vi "Dashboard Main.vi"() -> ()   [LabVIEW 2016]
uses:
  Program Files/National Instruments/LabVIEW 2016/examples/FRC/roboRIO/Vision/2017 Vision Example/Vision Support Code/Camera Types.ctl
  <vilib>/Rock Robotics/Network Tables/NT Read Boolean.vi
  <vilib>/Rock Robotics/Network Tables/NT Write Number.vi
  <vilib>/Rock Robotics/Network Tables/NT Read Number.vi
  <vilib>/Utility/file.llb/Read Delimited Spreadsheet (DBL).vi
  <vilib>/Utility/file.llb/Write Delimited Spreadsheet (DBL).vi
  <vilib>/vision/NI_Vision_Development_Module.lvlib
panel:
  out "Original Image":T1(plugin-control)
  in  "Dashboard Tab":T2(tab)=enum."\"Fudge\" Variables"
  out "Trim Close":dbl=-1.0
  out "Trim Far":dbl=-1.0
  out "Have Gear?":bool
  out "Drive Mode":bool
  in  "Auto Selector":T3(ring)
  out "Aimed?":bool
  out "IR Distance":bool
  out "Mode":T4(ring)=enum."Auto Disabled"
  in  "Camera Name":string(combo)="No Camera Selection"
  out "Camera Info":cluster{"Mbps LED":bool, "Mbps":dbl, "fps":dbl} {"fps" format="%#.1g"; "Mbps" format="%#.1g"}
  in  "Camera Type":T5=enum."MS HD3000 square"
  in  "LED Color":T6={"Hue"={70.0, 130.0}, "Sat"={150.0, 255.0}, "Val"={100.0, 255.0}} {"Hue" scale=0.0..255.0 scale format="%#_3g"}
  in  "Annotate":bool=TRUE
  in  "Color Mode":u16(ring)=2 items=["RGB", "HSL", "HSV", "HSI"]
  in  "Particles":dbl=4.0
  in  "Score Cutoff %":dbl=75.0
  out "Qualified Particles":i32
  in  "Std Devs for Calibration":cluster{"H":dbl, "S":dbl, "V":dbl}={"H"=4.0, "S"=6.0, "V"=6.0}
  in  "Line Border":cluster{"Top":dbl, "Bottom":dbl}={"Top"=6.0, "Bottom"=1.0}
  in  "Camera Settings":T7={"Frame Rate"=30, "Compression"=30, "Size"=1, "DB Camera Config"=FALSE} {"Frame Rate" scale=1.0..30.0; "Compression" scale=100.0..-1.0; "Size" items=["640x480", "320x240", "160x120"]}
  out "Mask":T1(plugin-control)
  out "Results":T8 {"Score" format="%#_3g"; "Pixels"."Rectangle"."Numeric 5" format="%#_3g"; "Pixels"."Rectangle"."Numeric 3" format="%#_3g"; "Pixels"."Rectangle"."Numeric 2" format="%#_3g"; "Pixels"."Rectangle"."Numeric" format="%#_3g"; "Normalized"."Rectangle"."Numeric 5" format="%#_2g"; "Normalized"."Rectangle"."Numeric 3" format="%#_2g"; "Normalized"."Rectangle"."Numeric 2" format="%#_2g"; "Normalized"."Rectangle"."Numeric" format="%#_2g"; "Normalized"."Center"."?" format="%#_3g"; "Normalized"."Center"."?" format="%#_3g"; "Distance (ft)" format="%#_3g"}
  in  "Autoaim fast":dbl=0.25
  in  "Autoaim mid":dbl=0.2
  in  "Autoaim slow":dbl=0.19
  in  "FF B40":dbl=0.7
  in  "B40yDepth":dbl=62.0
  in  "center gear depth":dbl=31.0
  in  "FF B10 G":dbl=0.72
  in  "FF R60 P1":dbl=0.71
  in  "FF R60 P2":dbl=0.704
  in  "Hopper Close":dbl=0.6
  in  "Hopper Far":dbl=0.75
  in  "R60P2yDepth":dbl=-74.0
  in  "R60P1yDepth":dbl=-60.0
  in  "Camera Target":dbl=0.06
  in  "FF Far Tele":dbl=0.7
  in  "FF Close Tele":dbl=0.66
  in  "Intake Speed":dbl=0.8
  out "Path":path
  out "Tree":string(tree)
  out "NT Connection":bool
  in  "Select Auto":string(combo)="Select Autonomous ..."
  out "Background":bool
  in  "TCP":refnum<k5>
  out "Robot IP":string
  out "Camera Image":T1(plugin-control)
  # "REALLY IMPORTANT"
  # "HW"
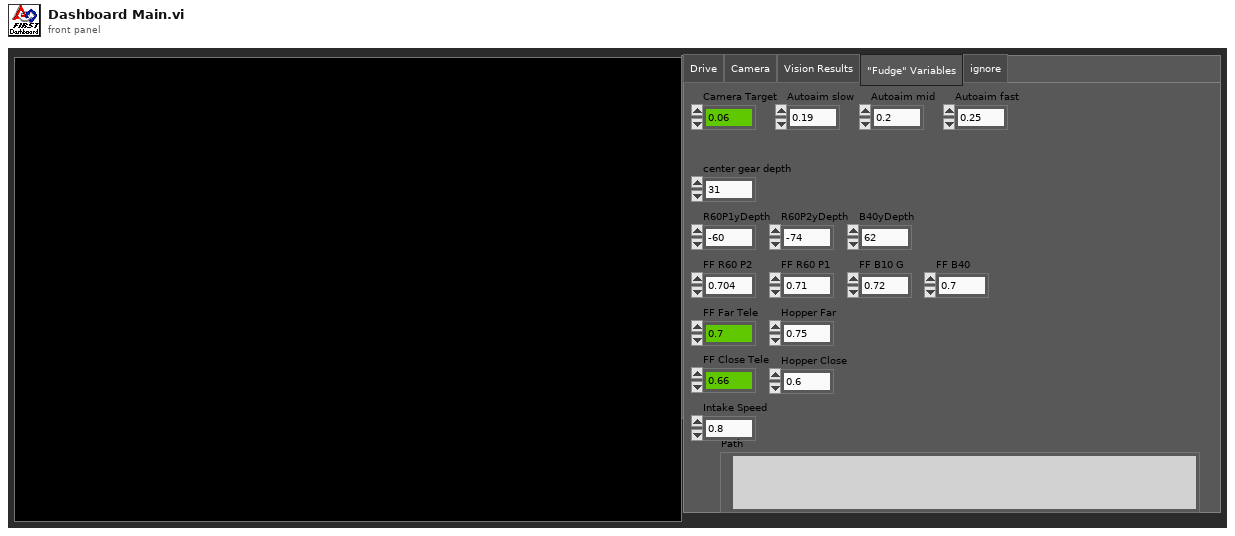
[diagram p1: front panel]
types:
  T1 = typedef "IMAQ Image.ctl" = refnum<image>
  T2 = enum32{"Drive", "Camera", "Vision Results", "\"Fudge\" Variables", "ignore"}
  T3 = enum16{"Do Nothing", "Blue 10 + Gear middle", "Red 10 + Gear middle", "Straight Gear", "Blue 40 P1", "Red 40 P1", "Red 40 P2", "Red 40 + Gear P2 (god auto DNE)", "Blue Side Gear P2 (unproven)"}
  T4 = enum8{"Tele-Op Disabled", "Tele-Op Enabled", "Auto Disabled", "Auto Enabled", "Test Disabled", "Test Enabled", "Disconnected", "No Code", "E-Stop"}
  T5 = typedef "Camera Types.ctl" = enum16{"206", "1011", "1013", "MS HD3000 square", "MS HD3000 640x480"}
  T6 = cluster{"Hue":cluster{dbl, dbl}, "Sat":cluster{dbl, dbl}, "Val":cluster{dbl, dbl}}
  T7 = cluster{"Frame Rate":i32, "Compression":i32, "Size":u16, "DB Camera Config":bool}
  T8 = cluster{"Distance (ft)":dbl, "Score":dbl, "Normalized":cluster{"Center":cluster{dbl, dbl}, "Rectangle":cluster{"Numeric":dbl, "Numeric 2":dbl, "Numeric 3":dbl, "Numeric 5":dbl}}, "Pixels":cluster{"Center":cluster{dbl, dbl}, "Rectangle":cluster{"Numeric":dbl, "Numeric 2":dbl, "Numeric 3":dbl, "Numeric 5":dbl}}}
  T9 = typedef "Particle Parameters" = i32
  T10 = typedef "Image Type" = u32
  T11 = enum32{"Drive", "Basic", "Custom", "Test", "Checklist", "Variables"}
  T12 = cluster{cluster{"Numeric":dbl, "Numeric":dbl}, cluster{"Numeric":dbl, "Numeric":dbl}, cluster{"Numeric":dbl, "Numeric":dbl}}
  T13 = cluster{"Camera Image":refnum<vi>, "Dashboard Tab":refnum<vi>, "Background":refnum<vi>, "Tree":refnum<vi>, "Camera Settings":refnum<vi>, "Camera Name":refnum<vi>, "Camera Info":refnum<vi>}
  T14 = cluster{"Error Strings":string, "Disable Counts":cluster{u16, u16}, "Rail Faults":cluster{u16, u16, u16}, "Robot IP":string, "DB Mode":u8, "Event Info":cluster{"Name":string, "Type":u8, "Number":u16, "Replay":u8}}
  T15 = cluster{"Storage":cluster{"Disk Free":u64, "RAM Block":u32, "RAM free":u32}, "CPU Utilization":cluster{"CPU % ISR":sgl, "CPU % Time Crit":sgl, "CPU % Timed Str":sgl, "CPU % High":sgl, "CPU % Above":sgl, "CPU % Normal":sgl, "CPU % Low":sgl}, "CAN":cluster{"% Bus Utilization":sgl, "Bus Off Cnt":u32, "TX_FIFO Full Cnt":u32, "Receive Error Cnt":u8, "Transmit Error Cnt":u8}, "HID":cluster{"HID Outputs":u32, "Rumble Low":u16, "Rumble High":u16}[]}
  T16 = cluster{"Status bits":cluster{"Test Mode":bool, "Autonomous":bool, "Enabled":bool, "Code Start":bool, "Brownout":bool, "Reserved 2":bool, "Reserved 3":bool, "E-Stop":bool}, "Code Trace":cluster{"Disabled":bool, "TeleOp":bool, "Auto":bool, "Test":bool}, "Controller Type":enum16{"unknown", "cRIO", "roboRio"}, "Code?":enum16{"unknown", "noCode", "code"}, "Battery V":dbl}
  T17 = cluster{"Control Bits":cluster{"TestMode":bool, "Autonomous":bool, "Enabled":bool, "FMS Present":bool, bool, bool, bool, "E-Stop":bool}, "Team Station ":u8, "Countdown":sgl, "Joystick Values":cluster{"Axes":dbl[], "Buttons":bool[], "POVs":i16[]}[]}
  T18 = cluster{"Shift":bool, "Ctrl":bool, "Alt":bool, "Cmd":bool, "Opt":bool}
  T19 = cluster{cluster{dbl, dbl}, cluster{dbl, dbl}, cluster{dbl, dbl}}
  T20 = cluster{"Left":dbl, "Top":dbl, "Right":dbl, "Bottom":dbl}
  T21 = cluster{"Center":cluster{dbl, dbl}, "Rectangle":cluster{"Numeric":dbl, "Numeric 2":dbl, "Numeric 3":dbl, "Numeric 5":dbl}}
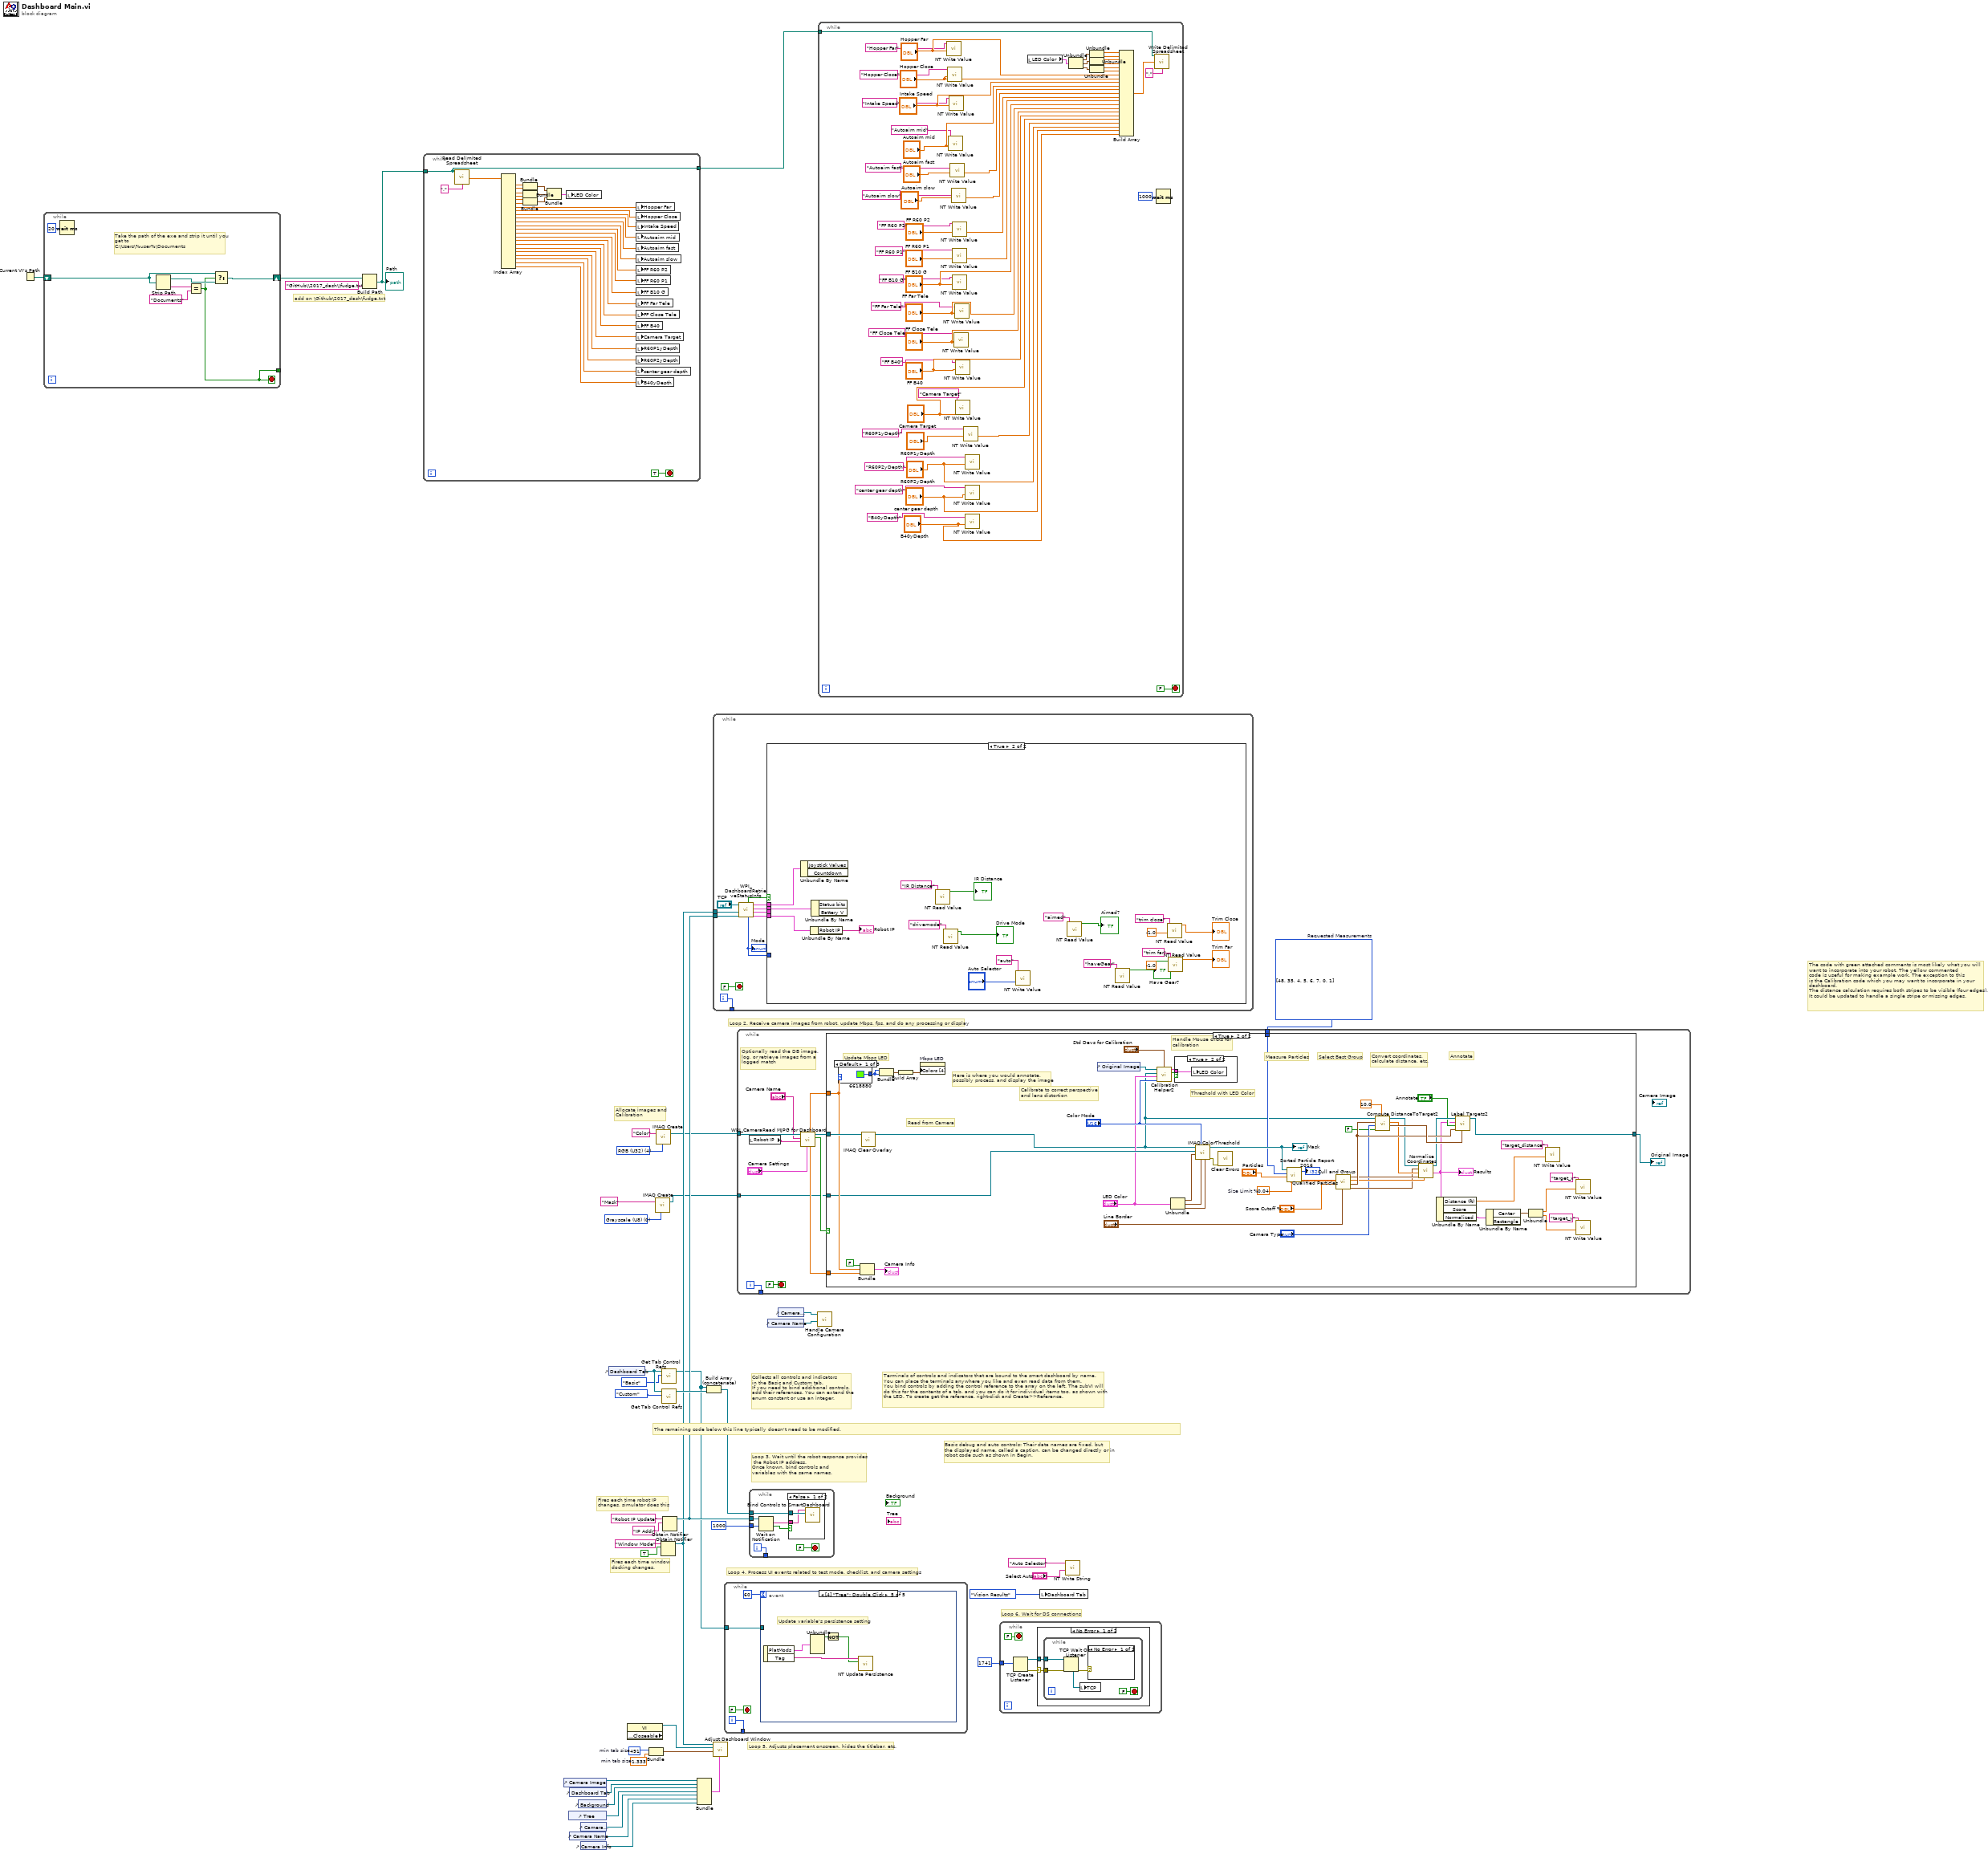
[diagram p0: block diagram]
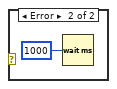
[diagram p2: hidden frame]
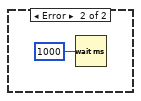
[diagram p3: hidden frame]
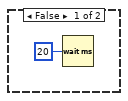
[diagram p4: hidden frame]
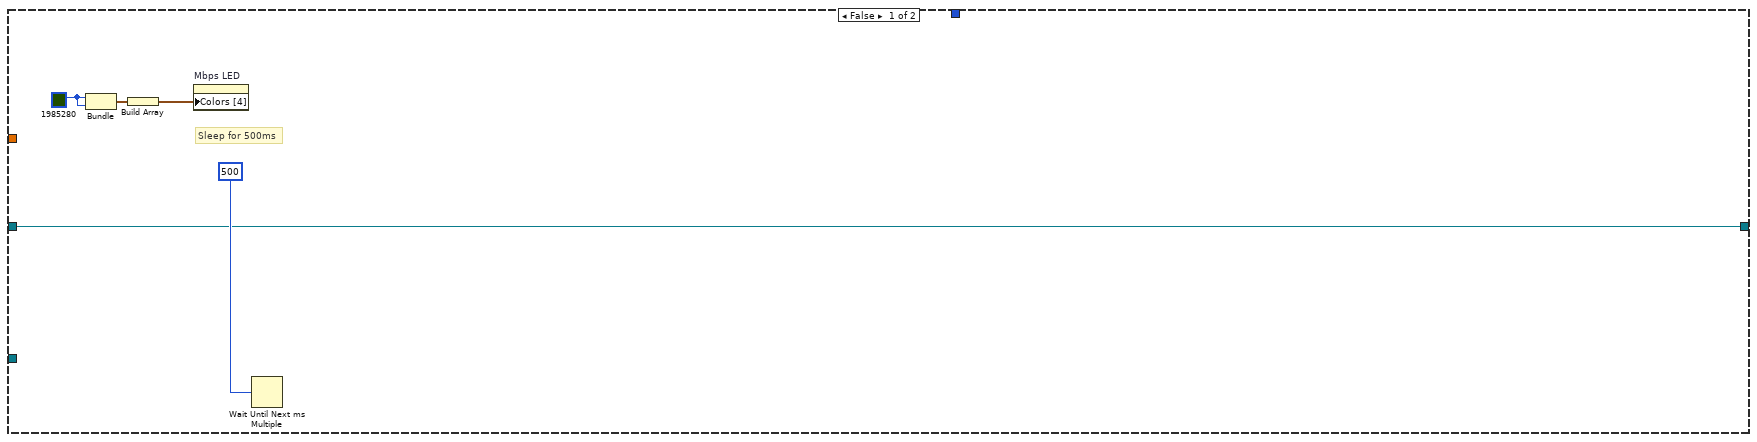
[diagram p6: hidden frame]
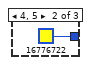
[diagram p8: hidden frame]
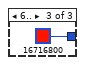
[diagram p9: hidden frame]
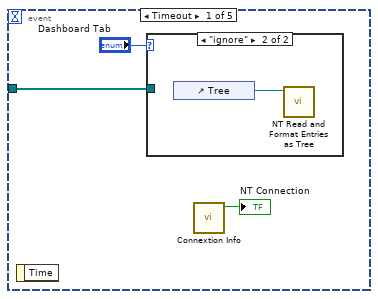
[diagram p10: hidden frame]
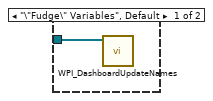
[diagram p11: hidden frame]
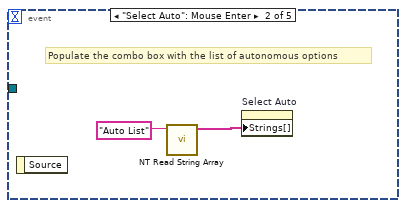
[diagram p12: hidden frame]
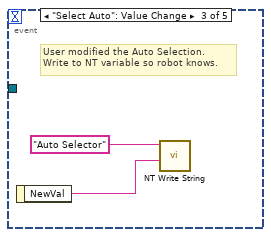
[diagram p13: hidden frame]
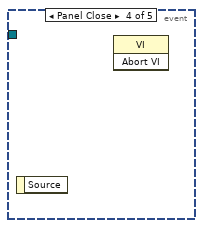
[diagram p14: hidden frame]
diagram:
  w6 = T9[] [48, 35, 4, 5, 6, 7, 0, 1] items=["Center of Mass X", "Center of Mass Y", "First Pixel X", "First Pixel Y", "Bounding Rect Left", "Bounding Rect Top", "Bounding Rect Right", "Bounding Rect Bottom", "Max Feret Diameter Start X", "Max Feret Diameter Start Y", "Max Feret Diameter End X", "Max Feret Diameter End Y", "Max Horiz. Segment Length Left", "Max Horiz. Segment Length Right", "Max Horiz. Segment Length Row", "-", "Bounding Rect Width", "Bounding Rect Height", "Bounding Rect Diagonal", "Perimeter", "Convex Hull Perimeter", "Holes' Perimeter", "Max Feret Diameter", "Equivalent Ellipse Major Axis", "Equivalent Ellipse Minor Axis", "Equivalent Ellipse Minor Axis (Feret)", "Equivalent Rect Long Side", "Equivalent Rect Short Side", "Equivalent Rect Diagonal", "Equivalent Rect Short Side (Feret)", "Average Horiz. Segment Length", "Average Vert. Segment Length", "Hydraulic Radius", "Waddel Disk Diameter", "-", "Area", "Holes' Area", "Particle & Holes' Area", "Convex Hull Area", "Image Area", "-", "Number of Holes", "Number of Horiz. Segments", "Number of Vert. Segments", "-", "Orientation", "Max Feret Diameter Orientation", "-", "% Area/Image Area", "% Area/(Particle & Holes' Area)", "Ratio of Equivalent Ellipse Axes", "Ratio of Equivalent Rect Sides", "-", "Elongation Factor", "Compactness Factor", "Heywood Circularity Factor", "Type Factor", "-", "Sum X", "Sum Y", "Sum XX", "Sum XY", "Sum YY", "Sum XXX", "Sum XXY", "Sum XYY", "Sum YYY", "-", "Moment of Inertia XX", "Moment of Inertia XY", "Moment of Inertia YY", "Moment of Inertia XXX", "Moment of Inertia XXY", "Moment of Inertia XYY", "Moment of Inertia YYY", "Norm. Moment of Inertia XX", "Norm. Moment of Inertia XY", "Norm. Moment of Inertia YY", "Norm. Moment of Inertia XXX", "Norm. Moment of Inertia XXY", "Norm. Moment of Inertia XYY", "Norm. Moment of Inertia YYY", "Hu Moment 1", "Hu Moment 2", "Hu Moment 3", "Hu Moment 4", "Hu Moment 5", "Hu Moment 6", "Hu Moment 7"]  # Requested Measurements
  w10 = T10 0 items=["Grayscale (U8)", "Grayscale (I16)", "Grayscale (SGL)", "Complex (CSG)", "RGB (U32)", "HSL (U32)", "RGB (U64)", "Grayscale (U16)"] ("Image Type")
  w11 = T10 4 items=["Grayscale (U8)", "Grayscale (I16)", "Grayscale (SGL)", "Complex (CSG)", "RGB (U32)", "HSL (U32)", "RGB (U64)", "Grayscale (U16)"] ("Image Type")
  w32 = 491  # min tab size
  w31 = 1.333  # min tab size
  # "add on \\Github\\2017_dash\\fudge.txt"
  # "The code with green attached comments is most likely what you will\nwant to incorporate into your robot. The yellow commented\ncode is useful for making example work. The exception to this\nis the Calibration code which you may want to incorporate in your\ndashboard.\nThe distance calculation requires both stripes to be visible (four edges).\nIt could be updated to handle a single stripe or missing edges."
  # "Allocate images and\nCalibration"
  # "Loop 6. Wait for DS connections"
  # "Basic debug and auto controls: Their data names are fixed, but\nthe displayed name, called a caption, can be changed directly or in\nrobot code such as shown in Begin."
  # "Fires each time robot IP\nchanges, simulator does this"
  # "Fires each time window\ndocking changes."
  # "Collects all controls and indicators\nin the Basic and Custom tab.\nIf you need to bind additional controls,\nadd their references. You can extend the\nenum constant or use an integer."
  # "The remaining code below this line typically doesn't need to be modified."
  # "Loop 4. Process UI events related to test mode, checklist, and camera settings"
  # "Terminals of controls and indicators that are bound to the smart dashboard by name.\nYou can place the terminals anywhere you like and even read data from them.\nYou bind controls by adding the control reference to the array on the left. The subVI will\ndo this for the contents of a tab, and you can do it for individual items too, as shown with\nthe LED. To create get the reference, right-click and Create>>Reference."
  # "Loop 3. Wait until the robot response provides\n the Robot IP address.\nOnce known, bind controls and\nvariables with the same names."
  # "Loop 5. Adjusts placement onscreen, hides the titlebar, etc."
  # "Loop 2. Receive camera images from robot, update Mbps, fps, and do any processing or display"
  n1 = Current VI's Path() -> (path=w5:path)
  n2 = while {
    shift-right: [w45] -> w4
    shift-left: w5 -> [w46]
    tunnel: [w44] -> _
    stop <- w44 stop-if-true
    # "Take the path of the exe and strip it until you\nget to\nC:\\Users\\%user%\\Documents"
    n3 = Wait (ms)(milliseconds to wait=u32 20) -> ()  [unwired: 1 out]
    n4 = Strip Path(path=w46) -> (stripped path=w47:path, name=w49:string)
    n5 = Equal?(x=w49, y="Documents") -> (x = y?=w44:bool)
    n6 = Select(t=w46, s=w44, f=w47) -> (s? t:f=w45:path)
  }
  n7 = Build Path(base path=w4, name or relative path="GitHub\\2017_dash\\fudge.txt") -> (appended path=w2:path)
  "Path" <- w2
  n8 = while {
    tunnel: w2 -> [w81]
    tunnel: [w81] -> w1
    stop <- TRUE stop-if-true
    n9 = call-poly <vilib>:"Read Delimited Spreadsheet.vi"("file path (dialog if empty)"=w81, "delimiter (\\t)"="," ("delimiter (\\t)")) -> ("first row"=w80:dbl[])  [unwired: 8 in, 5 out]
    n10 = Index Array(array=w80) -> (element #1=w79:dbl, element #2=w78:dbl, element #3=w77:dbl, element #4=w76:dbl, element #5=w75:dbl, element #6=w74:dbl, element #7=w69:dbl, element #8=w68:dbl, element #9=w66:dbl, element #10=w65:dbl, element #11=w64:dbl, element #12=w63:dbl, element #13=w62:dbl, element #14=w61:dbl, element #15=w60:dbl, element #16=w59:dbl, element #17=w58:dbl, element #18=w57:dbl, element #19=w56:dbl, element #20=w55:dbl, element #21=w54:dbl, element #22=w53:dbl, element #23=w52:dbl)  [unwired: 23 in]
    n11 = Bundle("Numeric"=w79, "Numeric"=w78) -> (w73:cluster{"Numeric":dbl, "Numeric":dbl})  [unwired: 1 in]
    n12 = Bundle("Numeric"=w77, "Numeric"=w76) -> (w72:cluster{"Numeric":dbl, "Numeric":dbl})  [unwired: 1 in]
    n13 = Bundle("Numeric"=w75, "Numeric"=w74) -> (w71:cluster{"Numeric":dbl, "Numeric":dbl})  [unwired: 1 in]
    n14 = Bundle(w73, w72, w71) -> (w70:T12)  [unwired: 1 in]
    n15 = local write "LED Color"(w70) -> ()
    n16 = local write "Hopper Far"(w69) -> ()
    n17 = local write "Hopper Close"(w68) -> ()
    n18 = local write "Intake Speed"(w66) -> ()
    n19 = local write "Autoaim mid"(w65) -> ()
    n20 = local write "Autoaim fast"(w64) -> ()
    n21 = local write "Autoaim slow"(w63) -> ()
    n22 = local write "FF R60 P2"(w62) -> ()
    n23 = local write "FF R60 P1"(w61) -> ()
    n24 = local write "FF B10 G"(w60) -> ()
    n25 = local write "FF Far Tele"(w59) -> ()
    n26 = local write "FF Close Tele"(w58) -> ()
    n27 = local write "FF B40"(w57) -> ()
    n28 = local write "Camera Target"(w56) -> ()
    n29 = local write "R60P1yDepth"(w55) -> ()
    n30 = local write "R60P2yDepth"(w54) -> ()
    n31 = local write "center gear depth"(w53) -> ()
    n32 = local write "B40yDepth"(w52) -> ()
  }
  n33 = control-ref of="Camera Image"() -> (w34:refnum<vi>)
  n34 = control-ref of="Tree"() -> (w16:refnum<vi>)
  n35 = control-ref of="Dashboard Tab"() -> (w33:refnum<vi>)
  n36 = control-ref of="Camera Name"() -> (w14:refnum<vi>)
  n37 = control-ref of="Background"() -> (w29:refnum<vi>)
  n38 = control-ref of="Camera Settings"() -> (w15:refnum<vi>)
  n39 = control-ref of="Camera Info"() -> (w13:refnum<vi>)
  n40 = control-ref of="Dashboard Tab"() -> (w37:refnum<vi>)
  n41 = property class="VI" props=["Front Panel.Closeable"]() -> (reference out=w38:refnum<vi>)  [unwired: 2 in, 2 out]
  n42 = Bundle("min tab size"=w32, "min tab size"=w31) -> (w30:cluster{"min tab size":i32, "min tab size":dbl})  [unwired: 1 in]
  n43 = call "IMAQ Create"("Image Name"="Mask", "Image Type"=w10) -> ("New Image"=w7:T1)  [unwired: 2 in, 2 out]
  n44 = call "IMAQ Create"("Image Name"="Color", "Image Type"=w11) -> ("New Image"=w8:T1)  [unwired: 2 in, 2 out]
  n45 = Obtain Notifier(name (unnamed)="Window Mode", notification data type=TRUE) -> (notifier out=w24:refnum<notifier>)  [unwired: 2 in, 2 out]
  n46 = call <vilib>:"Get Tab Control Refs.vi"("Page Index"=T11."Basic" ("Dashboard Tab"), "TabControl in"=w37) -> ("ControlsOnPage"=w19:refnum<vi>[])  [unwired: 9 in]
  n47 = call <vilib>:"Get Tab Control Refs.vi"("Page Index"=T11."Custom" ("Dashboard Tab"), "TabControl in"=w37) -> ("ControlsOnPage"=w36:refnum<vi>[])  [unwired: 9 in]
  n48 = Obtain Notifier(name (unnamed)="Robot IP Update", notification data type="IP Addr" ("name (unnamed)")) -> (notifier out=w25:refnum<notifier>)  [unwired: 2 in, 2 out]
  n49 = Bundle("Camera Image"=w34, "Dashboard Tab"=w33, "Background"=w29, "Tree"=w16, "Camera Settings"=w15, "Camera Name"=w14, "Camera Info"=w13) -> (w26:T13)  [unwired: 1 in]
  n50 = Build Array (concatenate)(w19, w36) -> (w35:refnum<vi>[])
  n51 = while {
    tunnel: [w91] -> _
    tunnel: w25 -> [w85]
    tunnel: w24 -> [w82]
    i -> [w91]
    stop <- FALSE stop-if-true
    n52 = call <vilib>:"WPI_DashboardRetrieveStatusInfo.vi"("Binding Refnum"=w85, "Window Mode Notifier"=w82, "TCP Cnx"="TCP") -> ("Power and Errors"=w86:T14, "Robot Metrics"=w89:T15, "Status Info"=w90:T16, "Control Info"=w87:T17, "Robot Mode"=w84:T4, "Process?"=w88:bool)  [unwired: 3 in]
    "Mode" <- w84
    n53 = case shown="True" w88 {
      tunnel: w90 -> [_ w113]
      tunnel: w89 -> [_ _]
      tunnel: w87 -> [_ w112]
      tunnel: w86 -> [_ w111]
      tunnel: w84 -> [_ _]
      frame False {
        n54 = Wait (ms)(milliseconds to wait=u32 20) -> ()  [unwired: 1 out]
      }
      frame True {
        n55 = Unbundle By Name(w112) -> ()  [unwired: 2 out]
        n56 = Unbundle By Name(w111) -> ("Robot IP"=→"Robot IP":string)
        n57 = Unbundle By Name(w113) -> ()  [unwired: 2 out]
        n58 = call-poly <vilib>:"NT Read Value.vi"("Name"="IR Distance") -> ("Boolean"=→"IR Distance":bool)  [unwired: 9 in, 1 out]
        n59 = call-poly <vilib>:"NT Read Value.vi"("Name"="drivemode") -> ("Boolean"=→"Drive Mode":bool)  [unwired: 9 in, 1 out]
        n60 = call-poly <vilib>:"NT Write Value.vi"("Numeric"="Auto Selector", "Name"="auto") -> ()  [unwired: 9 in, 1 out]
        n61 = call-poly <vilib>:"NT Read Value.vi"("Name"="aimed") -> ("Boolean"=→"Aimed?":bool)  [unwired: 9 in, 1 out]
        n62 = call-poly <vilib>:"NT Read Value.vi"("Name"="haveGear") -> ("Boolean"=→"Have Gear?":bool)  [unwired: 9 in, 1 out]
        n63 = call-poly <vilib>:"NT Read Value.vi"("Default Value"=-1.0, "Name"="trim close") -> ("Numeric"=→"Trim Close":dbl)  [unwired: 8 in, 1 out]
        n64 = call-poly <vilib>:"NT Read Value.vi"("Default Value"=-1.0, "Name"="trim far") -> ("Numeric"=→"Trim Far":dbl)  [unwired: 8 in, 1 out]
      }
    }
  }
  n65 = call "Adjust Dashboard Window.vi"("Sizing Refnums"=w26, "Size Constraints"=w30, "VI"=w38, "WIn Mode"=w24) -> ()  [unwired: 8 in]
  n66 = while {
    tunnel: [w115] -> _
    tunnel: w19 -> [w114]
    i -> [w115]
    stop <- FALSE stop-if-true
    n67 = event shown="[4] \"Tree\": Double Click" {
      selector: _ -> [_ _ _ _ _]
      dyn-events: _ -> [_ _ _ _ _]
      timeout: u32 60 ("milliseconds to wait") -> [_ _ _ _ _]
      tunnel: w114 -> [w118 _ _ _ _]
      event Timeout {
        n68 = event-data() -> ()  [unwired: 1 in, 1 out]
        n69 = case shown="\"ignore\"" "Dashboard Tab" {
          tunnel: w118 -> [w121 _]
          frame "\"Fudge\" Variables", Default {
            n70 = call <vilib>:"WPI_DashboardUpdateNames.vi"("Controls on Tab"=w121) -> ()  [unwired: 11 in]
          }
          frame "ignore" {
            n71 = control-ref of="Tree"() -> (w122:refnum<vi>)
            n72 = call <vilib>:"NT Read and Format Entries as Tree.vi"("Tree Refnum"=w122) -> ()  [unwired: 9 in, 2 out]
          }
        }
        n73 = call <vilib>:"Connextion Info.vi"() -> ("Connected"=→"NT Connection":bool)  [unwired: 10 in, 1 out]
      }
      event "Select Auto": Mouse Enter {
        # "Populate the combo box with the list of autonomous options"
        n74 = event-data() -> ()  [unwired: 1 in, 1 out]
        n75 = call <vilib>:"NT Read String Array.vi"("Name"="Auto List") -> ("String Array"=w123:string[])  [unwired: 9 in, 1 out]
        n76 = property on="Select Auto" class="CmbBox"("Strings[]"=w123) -> ()  [unwired: 2 in, 2 out]
      }
      event "Select Auto": Value Change {
        # "User modified the Auto Selection.\nWrite to NT variable so robot knows."
        n77 = event-data() -> ("NewVal"=w125:string)  [unwired: 1 in]
        n78 = call <vilib>:"NT Write String.vi"("String"=w125, "Name"="Auto Selector") -> ()  [unwired: 9 in, 1 out]
      }
      event Panel Close {
        n79 = event-data() -> ()  [unwired: 1 in, 1 out]
        n80 = invoke class="VI" method="Abort VI"() -> ()  [unwired: 3 in, 3 out]
      }
      event "Tree": Double Click {
        # "Update variable's persistence setting"
        n81 = event-data() -> ("PlatMods"=w130:T18, "Tag"=w129:string)  [unwired: 1 in]
        n82 = Unbundle(w130) -> ("Shift"=w128:bool)  [unwired: 4 out]
        n83 = Not(x=w128) -> (.not. x?=w127:bool)
        n84 = call <vilib>:"NT Update Persistence.vi"("Persistence"=w127, "Name"=w129) -> ()  [unwired: 9 in, 1 out]
      }
    }
  }
  n85 = while {
    tunnel: w8 -> [w141]
    tunnel: [w142] -> _
    tunnel: w7 -> [w133]
    tunnel: w6 -> [w131]
    i -> [w142]
    stop <- FALSE stop-if-true
    # "Optionally read the DB image,\nlog, or retrieve images from a\nlogged match"
    n86 = local read "Robot IP"() -> (w137:string)
    n87 = call <vilib>:"WPI_CameraRead MJPG for Dashboard.vi"("Camera Settings"="Camera Settings", "Robot IP"=w137, "Camera Name"="Camera Name", "Refnum in"=w141) -> ("Active"=w139:bool, "Refnum out"=w140:T1, "FPS"=w138:dbl, "Bandwidth (Mbps)"=w136:dbl)  [unwired: 4 in]
    n88 = case shown="True" w139 {
      tunnel: w140 -> [w144 w196]
      tunnel: w136 -> [_ w193]
      tunnel: w138 -> [_ w194]
      tunnel: [w144 w168] -> w132
      tunnel: w133 -> [_ w169]
      tunnel: w131 -> [_ w167]
      frame False {
        w146 = u32 1985280 ("Color Box")
        # "Sleep for 500ms"
        n89 = Bundle("Color Box"=w146, "Color Box"=w146) -> (w147:cluster{"Color Box":u32, "Color Box":u32})  [unwired: 1 out]
        n90 = Build Array(w147) -> (w145:cluster{"Color Box":u32, "Color Box":u32}[])
        n91 = property on="Mbps LED" class="Bool (strict)"("Colors [4]"=w145) -> ()  [unwired: 2 in, 2 out]
        n92 = Wait Until Next ms Multiple(millisecond multiple=u32 500) -> ()  [unwired: 1 out]
      }
      frame True {
        w174 = 0.04  # Size Limit %
        # "Read from Camera"
        # "Calibrate to correct perspective\nand lens distortion"
        # "Handle Mouse clicks for\ncalibration"
        # "Measure Particles"
        # "Convert coordinates,\ncalculate distance, etc."
        # "Annotate"
        # "Select Best Group"
        # "Threshold with LED Color"
        # "Here is where you would annotate,\npossibly process, and display the image"
        # "Update Mbps LED"
        n93 = case shown="Default" w193 {
          tunnel: [u32 6618880 ("Color Box") u32 16776722 ("Color Box") u32 16716800 ("Color Box")] -> w197
          frame Default {
          }
          frame 4, 5 {
          }
          frame 6.. {
          }
        }
        n94 = Bundle(FALSE, "Bandwidth (Mbps)"=w193, "FPS"=w194) -> (→"Camera Info":cluster{bool, "Bandwidth (Mbps)":dbl, "FPS":dbl})  [unwired: 1 in]
        n95 = call "IMAQ Clear Overlay"("Image"=w196) -> ("Image Out"=w153:T1)  [unwired: 2 in, 8 out]
        n96 = Bundle("Color Box"=w197, "Color Box"=w197) -> (w198:cluster{"Color Box":u32, "Color Box":u32})  [unwired: 1 out]
        n97 = Build Array(w198) -> (w195:cluster{"Color Box":u32, "Color Box":u32}[])
        n98 = property on="Mbps LED" class="Bool (strict)"("Colors [4]"=w195) -> ()  [unwired: 2 in, 2 out]
        n99 = control-ref of="Original Image"() -> (w152:refnum<vi>)
        n100 = call "Calibration Helper2.vi"("Std Devs"="Std Devs for Calibration", "Color Mode"="Color Mode", "Color Components"="LED Color", "Image"=w153, "Image Ctl Refnum"=w152) -> ("Changed"=w157:bool, "output color"=w158:T19)  [unwired: 5 in]
        n101 = Unbundle("LED Color") -> ("Hue"=w170:cluster{dbl, dbl}, "Sat"=w171:cluster{dbl, dbl}, "Val"=w172:cluster{dbl, dbl})
        n102 = case shown="True" w157 {
          tunnel: w158 -> [_ w199]
          frame False {
          }
          frame True {
            n103 = local write "LED Color"(w199) -> ()
          }
        }
        n104 = call "IMAQ ColorThreshold"("Blue or Luma or Val or Inten Range"=w172, "Green or Sat Range"=w171, "Color Mode"="Color Mode", "Red or Hue Range"=w170, "Image Dst"=w169, "Image Src"=w153) -> ("error out"=w176:errorcluster, "Image Dst Out"=w179:T1)  [unwired: 4 in]
        "Mask" <- w179
        n105 = call <vilib>:"Clear Errors.vi"("error in (no error)"=w176) -> ()  [unwired: 5 in, 2 out]
        n106 = call "Sorted Particle Report 2016.vi"("Min Area Size %"=w174, "Particle Count Limit"="Particles", "Pixel Measurements"=w167, "Image in"=w179) -> ("Sorted Data"=w177:dbl[][], "Particles"=→"Qualified Particles":i32)
        n107 = call "Cull and Group.vi"("Line Border"="Line Border", "Score Cutoff"="Score Cutoff %", "Sorted Data"=w177) -> ("Rect"=w181:T20, "Line"=w188:T20, "Score"=w186:dbl, "Center"=w185:cluster{"X":dbl, "Y":dbl})  [unwired: 5 in]
        n108 = call "Compute DistanceToTarget2.vi"("Fudge Dist Num"=10.0, "Calibrated"=FALSE, "Camera Type"="Camera Type", "Line"=w188, "Image Src"=w153) -> ("Edges"=w189:cluster{"X":sgl, "Y":sgl}[], "Distance (ft)"=w182:dbl, "Image Dst Out"=w183:T1)  [unwired: 4 in]
        n109 = call "Normalize Coordinates.vi"("Score"=w186, "Center"=w185, "Distance"=w182, "Bounding box"=w181, "Image in"=w183) -> ("Results"=w166:T8, "Image out"=w184:T1)  [unwired: 5 in]
        "Results" <- w166
        n110 = Unbundle By Name(w166) -> ("Distance (ft)"=w150:dbl, "Normalized"=w165:T21)  [unwired: 1 out]
        n111 = call "Label Targets2.vi"("Edges"=w189, "Line"=w188, "Annotate"="Annotate", "Results"=w166, "Image in"=w184) -> ("Image out"=w168:T1)  [unwired: 6 in]
        n112 = Unbundle By Name(w165) -> ("Center"=w162:cluster{dbl, dbl})  [unwired: 1 out]
        n113 = Unbundle(w162) -> (w161:dbl, w160:dbl)
        n114 = call-poly <vilib>:"NT Write Value.vi"("Numeric"=w150, "Name"="target_distance") -> ()  [unwired: 9 in, 1 out]
        n115 = call-poly <vilib>:"NT Write Value.vi"("Numeric"=w161, "Name"="target_x") -> ()  [unwired: 9 in, 1 out]
        n116 = call-poly <vilib>:"NT Write Value.vi"("Numeric"=w160, "Name"="target_y") -> ()  [unwired: 9 in, 1 out]
      }
    }
    "Original Image" <- w132
  }
  n117 = while {
    tunnel: w35 -> [w209]
    tunnel: w25 -> [w207]
    tunnel: [w205] -> _
    tunnel: u32 1000 ("milliseconds to wait") -> [w204]
    i -> [w205]
    stop <- FALSE stop-if-true
    n118 = Wait on Notification(notifier=w207, timeout in ms (-1)=w204) -> (notification=w206:string, timed out?=w203:bool)  [unwired: 2 in, 2 out]
    n119 = case shown="False" w203 {
      tunnel: w209 -> [w211 _]
      tunnel: w206 -> [w210 _]
      frame False {
        n120 = call <vilib>:"Bind Controls to SmartDashboard.vi"("Bound Control Refs"=w211, "Server IP Address"=w210) -> ()  [unwired: 10 in]
      }
      frame True {
      }
    }
  }
  n121 = control-ref of="Camera Name"() -> (w20:refnum<vi>)
  n122 = control-ref of="Camera Settings"() -> (w21:refnum<vi>)
  n123 = call "Handle Camera Configuration.vi"("CameraNameRef"=w20, "ClusterRef"=w21) -> ()  [unwired: 10 in]
  n124 = while {
    tunnel: w1 -> [w215]
    stop <- FALSE stop-if-true
    n125 = call-poly <vilib>:"NT Write Value.vi"("Numeric"="Hopper Far", "Name"="Hopper Far") -> ()  [unwired: 9 in, 1 out]
    n126 = call-poly <vilib>:"NT Write Value.vi"("Numeric"="Hopper Close", "Name"="Hopper Close") -> ()  [unwired: 9 in, 1 out]
    n127 = call-poly <vilib>:"NT Write Value.vi"("Numeric"="Autoaim mid", "Name"="Autoaim mid") -> ()  [unwired: 9 in, 1 out]
    n128 = call-poly <vilib>:"NT Write Value.vi"("Numeric"="Intake Speed", "Name"="Intake Speed") -> ()  [unwired: 9 in, 1 out]
    n129 = call-poly <vilib>:"NT Write Value.vi"("Numeric"="Autoaim fast", "Name"="Autoaim fast") -> ()  [unwired: 9 in, 1 out]
    n130 = call-poly <vilib>:"NT Write Value.vi"("Numeric"="Autoaim slow", "Name"="Autoaim slow") -> ()  [unwired: 9 in, 1 out]
    n131 = call-poly <vilib>:"NT Write Value.vi"("Numeric"="FF R60 P2", "Name"="FF R60 P2") -> ()  [unwired: 9 in, 1 out]
    n132 = call-poly <vilib>:"NT Write Value.vi"("Numeric"="FF R60 P1", "Name"="FF R60 P1") -> ()  [unwired: 9 in, 1 out]
    n133 = call-poly <vilib>:"NT Write Value.vi"("Numeric"="FF B10 G", "Name"="FF B10 G") -> ()  [unwired: 9 in, 1 out]
    n134 = call-poly <vilib>:"NT Write Value.vi"("Numeric"="FF Close Tele", "Name"="FF Close Tele") -> ()  [unwired: 9 in, 1 out]
    n135 = call-poly <vilib>:"NT Write Value.vi"("Numeric"="FF Far Tele", "Name"="FF Far Tele") -> ()  [unwired: 9 in, 1 out]
    n136 = call-poly <vilib>:"NT Write Value.vi"("Numeric"="FF B40", "Name"="FF B40") -> ()  [unwired: 9 in, 1 out]
    n137 = call-poly <vilib>:"NT Write Value.vi"("Numeric"="Camera Target", "Name"="Camera Target") -> ()  [unwired: 9 in, 1 out]
    n138 = call-poly <vilib>:"NT Write Value.vi"("Numeric"="R60P1yDepth", "Name"="R60P1yDepth") -> ()  [unwired: 9 in, 1 out]
    n139 = call-poly <vilib>:"NT Write Value.vi"("Numeric"="R60P2yDepth", "Name"="R60P2yDepth") -> ()  [unwired: 9 in, 1 out]
    n140 = call-poly <vilib>:"NT Write Value.vi"("Numeric"="center gear depth", "Name"="center gear depth") -> ()  [unwired: 9 in, 1 out]
    n141 = call-poly <vilib>:"NT Write Value.vi"("Numeric"="B40yDepth", "Name"="B40yDepth") -> ()  [unwired: 9 in, 1 out]
    n142 = local read "LED Color"() -> (w243:T6)
    n143 = Unbundle(w243) -> ("Hue"=w239:cluster{dbl, dbl}, "Sat"=w240:cluster{dbl, dbl}, "Val"=w241:cluster{dbl, dbl})
    n144 = Unbundle(w239) -> (w233:dbl, w234:dbl)
    n145 = Unbundle(w240) -> (w235:dbl, w236:dbl)
    n146 = Unbundle(w241) -> (w237:dbl, w238:dbl)
    n147 = Build Array(w233, w234, w235, w236, w237, w238, "Hopper Far", "Hopper Close", "Intake Speed", "Autoaim mid", "Autoaim fast", "Autoaim slow", "FF R60 P2", "FF R60 P1", "FF B10 G", "FF Far Tele", "FF Close Tele", "FF B40", "Camera Target", "R60P1yDepth", "R60P2yDepth", "center gear depth", "B40yDepth") -> (w242:dbl[])
    n148 = call-poly <vilib>:"Write Delimited Spreadsheet.vi"("file path (dialog if empty)"=w215, "1D data"=w242, "delimiter (\\t)"="," ("delimiter (\\t)")) -> ()  [unwired: 11 in, 2 out]
    n149 = Wait (ms)(milliseconds to wait=u32 1000) -> ()  [unwired: 1 out]
  }
  n150 = while {
    tunnel: u16 1741 ("timeout ms (25000)") -> [w262]
    stop <- FALSE stop-if-true
    n151 = TCP Create Listener(10:w262) -> (0:w261:errorcluster, 3:w263:refnum<k5>)  [unwired: 4 in, 1 out]
    n152 = case shown="No Error" w261 {
      selector: w261 -> [w265 _]
      tunnel: w263 -> [w266 _]
      frame No Error {
        n153 = while {
          tunnel: w266 -> [w269]
          tunnel: w265 -> [w268]
          stop <- FALSE stop-if-true
          n154 = TCP Wait On Listener(8:w268, 11:w269) -> (0:w270:errorcluster, 4:w271:refnum<k5>)  [unwired: 2 in, 3 out]
          n155 = local write "TCP"(w271) -> ()
          n156 = case shown="No Error" w270 {
            frame No Error {
            }
            frame Error {
              n157 = Wait (ms)(milliseconds to wait=u32 1000) -> ()  [unwired: 1 out]
            }
          }
        }
      }
      frame Error {
        n158 = Wait (ms)(milliseconds to wait=u32 1000) -> ()  [unwired: 1 out]
      }
    }
  }
  n159 = local write "Dashboard Tab"(T2."Vision Results" ("Dashboard Tab")) -> ()
  n160 = call <vilib>:"NT Write String.vi"("String"="Select Auto", "Name"="Auto Selector") -> ()  [unwired: 9 in, 1 out]
